vi "Init.vi"(8 "error in (no error)":errorcluster, 9 "Config File Path":path=path "", 10 "Name":string, 11 "Process In":refnum<class "Mock Debug Message Receiver.lvclass">) -> (0 "error out":errorcluster, 3 "Process Out":refnum<class "Mock Debug Message Receiver.lvclass">)   [LabVIEW 2020, in "Mock Debug Message Receiver.lvclass"]
doc: "Initializes the process and creates necessary references. Anything initialized here is released in the Clear.vi method."
uses:
  Mock Debug Message Receiver.lvclass
  Debug Message Receiver/Public/Debug Data Cluster.ctl
  Mock Debug Message Receiver.lvclass/Mock Debug Message Receiver.ctl
  Process/Debug Process.lvclass
  Debug Data Event/Debug Data Event.lvclass
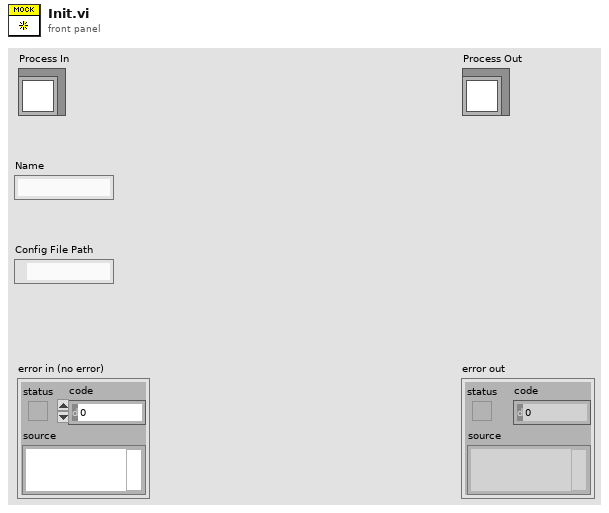
[diagram p1: front panel]
types:
  T1 = cluster{"Action":string, "Call Chain":string, "Process":string, "Message":string, "Message Data":variant, "Time":u32}
  T2 = typedef "Debug Data Event.lvclass/Debug Data Cluster.ctl" = cluster{"Action":string, "Call Chain":string, "Process":string, "Message":string, "Message Data":variant, "Time":u32}
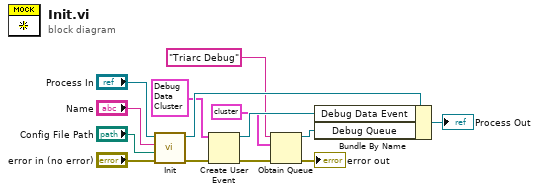
[diagram p0: block diagram]
diagram:
  n1 = call-parent "Init.vi"("error in (no error)"="error in (no error)", "Config File Path"="Config File Path", "Name"="Name", "Process In"="Process In") -> ("error out"=w8:errorcluster, "Process Out"=w14:refnum<class "Mock Debug Message Receiver.lvclass">)  [unwired: 6 in]
  n2 = Create User Event(user event datatype=T2 {"Action"="", "Call Chain"="", "Process"="", "Message"="", "Message Data"=variant, "Time"=0} ("Debug Data Cluster"), error in=w8) -> (user event=w6:refnum<user-event>, error out=w3:errorcluster)
  n3 = Obtain Queue(name (unnamed)="Triarc Debug", element data type=T1 {"Action"="", "Call Chain"="", "Process"="", "Message"="", "Message Data"=variant, "Time"=0} ("output cluster"), error in (no error)=w3) -> (queue out=w1:refnum<queue>, error out=→"error out":errorcluster)  [unwired: 2 in, 1 out]
  n4 = Bundle By Name(cluster=w14, "Debug Data Event"=w6, "Debug Queue"=w1) -> (→"Process Out":refnum<class "Mock Debug Message Receiver.lvclass">)
